vi "Create and Run Script.vi"(5 "Script Steps":string="generate HV29", 8 "Error In":errorcluster, 11 "HSDIO Sessions":T1) -> (0 "Error Out":errorcluster)   [LabVIEW 2013]
uses:
  <instrlib>/niHSDIO/niHSDIO.llb/niHSDIO_ctl Generation Mode Values (Ring).ctl
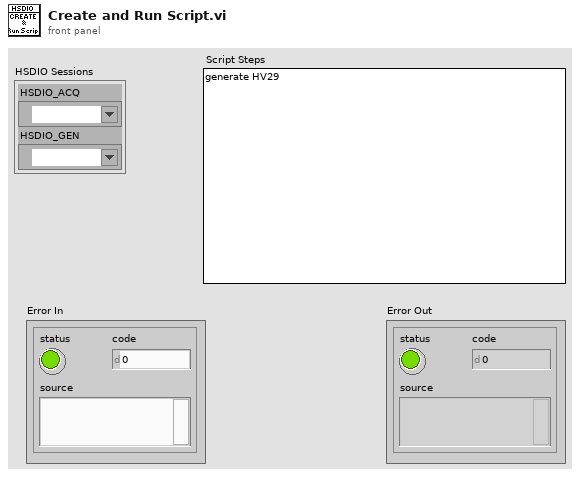
[diagram p1: front panel]
types:
  T1 = cluster{"HSDIO_ACQ":refnum<k15>, "HSDIO_GEN":refnum<k15>}
  T2 = typedef "niHSDIO_ctl Generation Mode Values (Ring).ctl" = i32
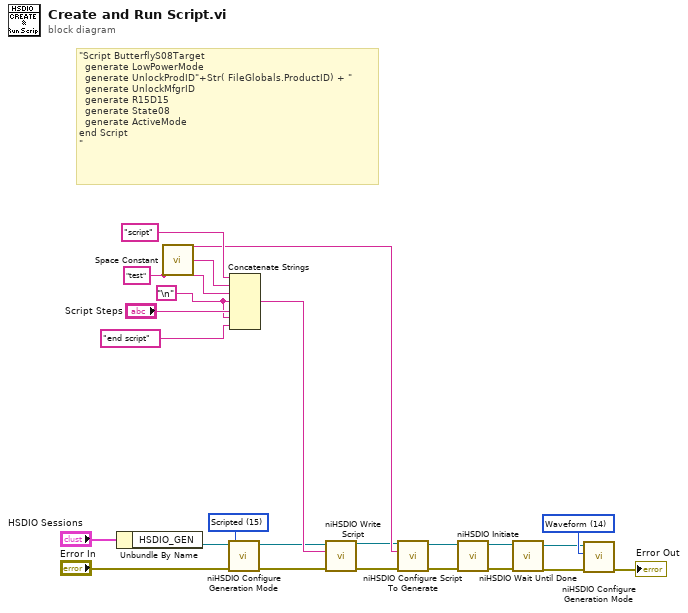
[diagram p0: block diagram]
diagram:
  w20 = "test" ("Script Name")
  w13 = T2 14 items=["Waveform"=14, "Scripted"=15] ("generation mode (waveform)")
  w14 = T2 15 items=["Waveform"=14, "Scripted"=15] ("generation mode (waveform)")
  w16 = "\n"
  # "\"Script ButterflyS08Target\n  generate LowPowerMode\n  generate UnlockProdID\"+Str( FileGlobals.ProductID) + \"\n  generate UnlockMfgrID\n  generate R15D15\n  generate State08\n  generate ActiveMode\nend Script\n\""
  n1 = Unbundle By Name("HSDIO Sessions") -> ("HSDIO_GEN"=w3:refnum<k15>)
  n2 = call <vilib>:"Space Constant.vi"() -> ("String"=w22:string)
  n3 = call <instrlib>:"niHSDIO Configure Generation Mode.vi"("error in (no error)"="Error In", "generation mode (waveform)"=w14, "instrument handle"=w3) -> ("error out"=w12:errorcluster, "instrument handle out"=w11:refnum<k15>)  [unwired: 7 in]
  n4 = Concatenate Strings("script" ("string"), w22, w20, w16, "Script Steps", w16, "end script") -> (w18:string)
  n5 = call <instrlib>:"niHSDIO Write Script.vi"("error in (no error)"=w12, "script"=w18, "instrument handle"=w11) -> ("error out"=w21:errorcluster, "instrument handle out"=w19:refnum<k15>)  [unwired: 7 in]
  n6 = call <instrlib>:"niHSDIO Configure Script To Generate.vi"("error in (no error)"=w21, "script name"=w20, "instrument handle"=w19) -> ("error out"=w7:errorcluster, "instrument handle out"=w8:refnum<k15>)  [unwired: 7 in]
  n7 = call <instrlib>:"niHSDIO Initiate.vi"("error in (no error)"=w7, "instrument handle"=w8) -> ("error out"=w10:errorcluster, "instrument handle out"=w9:refnum<k15>)  [unwired: 8 in]
  n8 = call <instrlib>:"niHSDIO Wait Until Done.vi"("error in (no error)"=w10, "instrument handle"=w9) -> ("error out"=w6:errorcluster, "instrument handle out"=w5:refnum<k15>)  [unwired: 8 in]
  n9 = call <instrlib>:"niHSDIO Configure Generation Mode.vi"("error in (no error)"=w6, "generation mode (waveform)"=w13, "instrument handle"=w5) -> ("error out"=→"Error Out":errorcluster)  [unwired: 7 in, 1 out]
